vi "Replace SubFunctions.vi"(0 "Function String":string, 11 "error in (no error)":errorcluster) -> (4 "Replace Sub Function with variable":string, 6 "Sub Functions":string[](array[string]), 8 "Variables":string[](array[string]), 15 "error out":errorcluster)   [LabVIEW 2019]
panel:
  # "(aaa)\n(aa + (bb))\n(aa * (ee)) + (bb) - cc * (dd)"
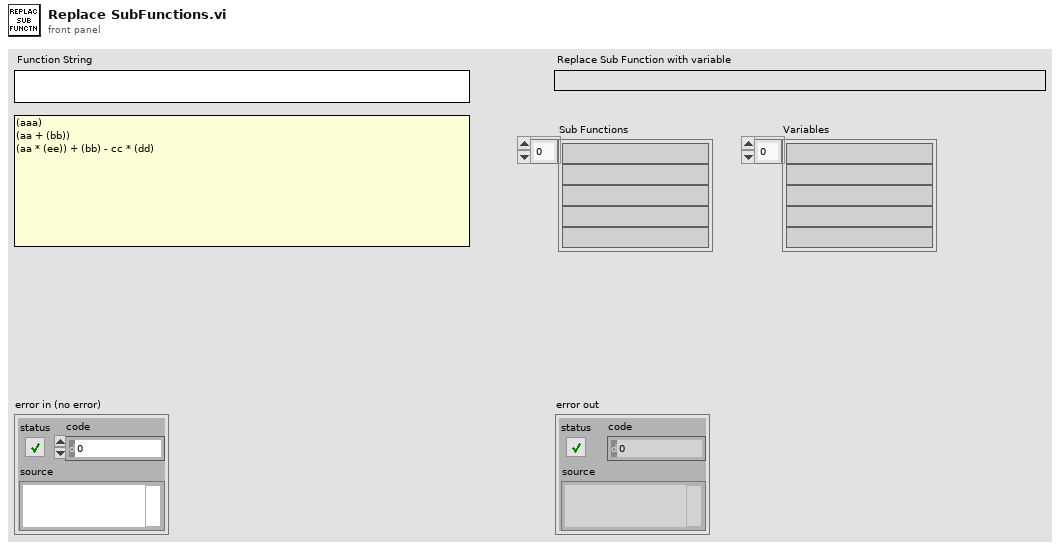
[diagram p1: front panel]
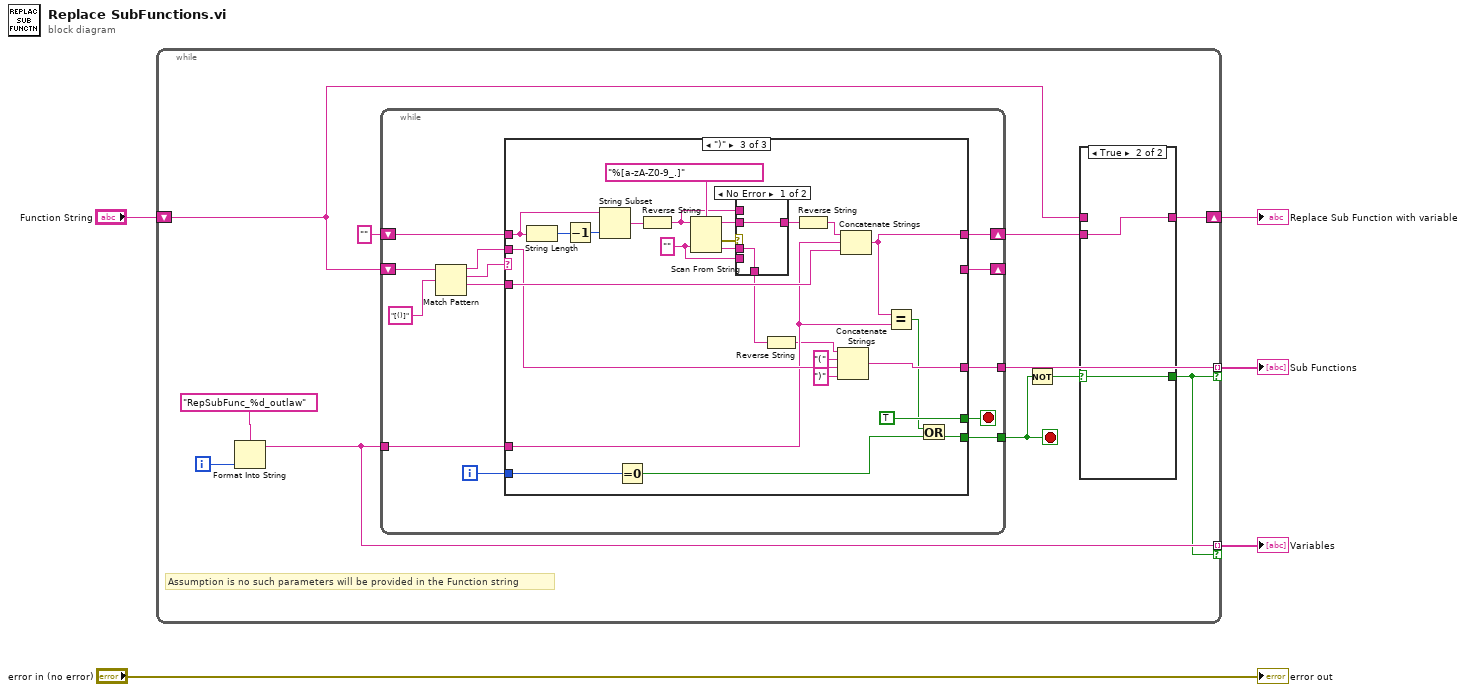
[diagram p0: block diagram]
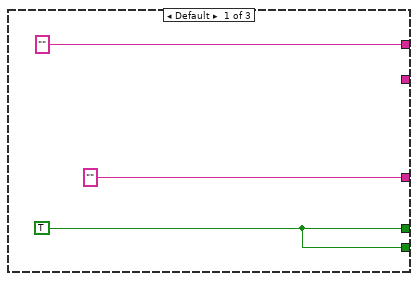
[diagram p3: hidden frame]
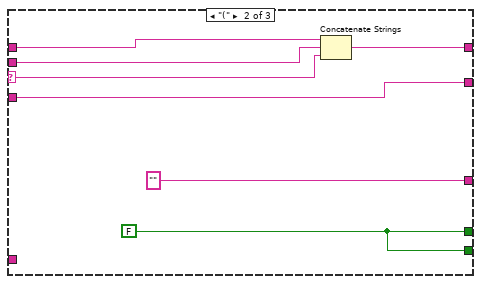
[diagram p4: hidden frame]
diagram:
  n1 = while {
    tunnel: [w16] -> w2 mode=indexing if=w7
    tunnel: [w8] -> w1 mode=indexing if=w7
    shift-right: [w13] -> w3
    shift-left: "Function String" -> [w12]
    i -> [w10]
    stop <- w15 stop-if-true
    # "Assumption is no such parameters will be provided in the Function string"
    n2 = Format Into String(format string="RepSubFunc_%d_outlaw", w10) -> (resulting string=w8:string)  [unwired: 2 in, 1 out]
    n3 = while {
      tunnel: [w29] -> w15
      shift-right: [w26] -> _
      shift-left: w12 -> [w25]
      tunnel: [w24] -> w16
      shift-right: [w28] -> w11
      shift-left: "" ("Function String") -> [w23]
      tunnel: w8 -> [w22]
      i -> [w21]
      stop <- w30 stop-if-true
      n4 = Match Pattern(string=w25, regular expression="[()]") -> (before substring=w31:string, match substring=w32:string, after substring=w27:string)  [unwired: 1 in, 1 out]
      n5 = case shown="\")\"" w32 {
        selector: w32 -> [_ w40 _]
        tunnel: w31 -> [_ w37 w67]
        tunnel: ["" ("Function String") w39 w58] -> w28
        tunnel: [w36 w42 TRUE] -> w30
        tunnel: [w36 w42 w56] -> w29
        tunnel: w27 -> [_ w43 w68]
        tunnel: [_ w43 _] -> w26
        tunnel: ["" "" w66] -> w24
        tunnel: w23 -> [_ w38 w60]
        tunnel: w22 -> [_ _ w57]
        tunnel: w21 -> [_ _ w63]
        frame Default {
          w36 = TRUE
        }
        frame "(" {
          w42 = FALSE
          n6 = Concatenate Strings(w38, w37, w40) -> (w39:string)
        }
        frame ")" {
          w44 = ""
          n7 = String Length(string=w60) -> (length=w61:i32)
          n8 = Decrement(x=w61) -> (x-1=w62:i32)
          n9 = String Subset(string=w60, length (rest)=w62) -> (substring=w54:string)  [unwired: 1 in]
          n10 = Equal To 0?(x=w63) -> (x = 0?=w59:bool)
          n11 = Reverse String(1:w54) -> (0:w45:string)
          n12 = Scan From String(format string="%[a-zA-Z0-9_.]", input string=w45, default 1=w44) -> (remaining string=w51:string, error out=w52:errorcluster, output 1=w50:string)  [unwired: 2 in, 1 out]
          n13 = case shown="No Error" w52 {
            tunnel: w51 -> [w70 _]
            tunnel: w50 -> [w71 _]
            tunnel: [w71 w72] -> w47
            tunnel: [w70 w73] -> w48
            tunnel: w45 -> [_ w73]
            tunnel: w44 -> [_ w72]
            frame No Error {
            }
            frame Error {
            }
          }
          n14 = Reverse String(1:w47) -> (0:w46:string)
          n15 = Reverse String(1:w48) -> (0:w49:string)
          n16 = Concatenate Strings(w46, "(" ("string"), w67, ")" ("string")) -> (w66:string)
          n17 = Concatenate Strings(w49, w57, w68) -> (w58:string)
          n18 = Equal?(x=w58, y=w57) -> (x = y?=w55:bool)
          n19 = Or(x=w55, y=w59) -> (x .or. y?=w56:bool)
        }
      }
    }
    n20 = Not(x=w15) -> (.not. x?=w14:bool)
    n21 = case shown="True" w14 {
      selector: w14 -> [w17 w20]
      tunnel: [w18 w19] -> w13
      tunnel: w12 -> [w18 _]
      tunnel: [w17 w20] -> w7
      tunnel: w11 -> [_ w19]
      frame False {
      }
      frame True {
      }
    }
  }
  "Replace Sub Function with variable" <- w3
  "Sub Functions" <- w2
  "Variables" <- w1
  "error out" <- "error in (no error)"
